vi "subVI for match count.vi"(10 "String":string="h*el*l*o**w*or*ld") -> (2 "Number of matches for \\n":dbl)   [LabVIEW 2012]
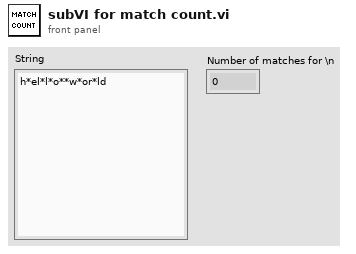
[diagram p1: front panel]
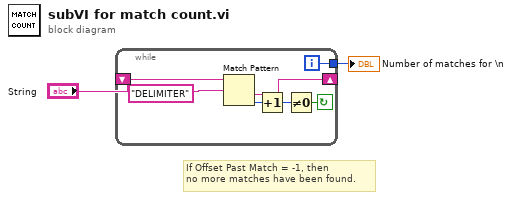
[diagram p0: block diagram]
diagram:
  # "If Offset Past Match = -1, then\nno more matches have been found."
  n1 = while {
    tunnel: [w4] -> w1
    shift-left: "String" -> [w9]
    shift-right: [w8] -> _
    i -> [w4]
    stop <- w5 continue-if-true
    n2 = Match Pattern(string=w9, regular expression="DELIMITER") -> (after substring=w8:string, offset past match=w7:i32)  [unwired: 1 in, 2 out]
    n3 = Increment(x=w7) -> (x+1=w6:i32)
    n4 = Not Equal To 0?(x=w6) -> (x != 0?=w5:bool)
  }
  "Number of matches for \\n" <- w1
